vi "Reshaper1.vi"(3 "error IN":errorcluster, 5 "[IN] (X,Y,dX,dY)":dbl[][](array[numeric])) -> (0 "error OUT":errorcluster, 2 "[OUT] Reshaped (X,Y,dX,dY)":dbl[][](array[numeric]))   [LabVIEW 2017]
doc: "Deleting zero points in tracks (zero displacements)"
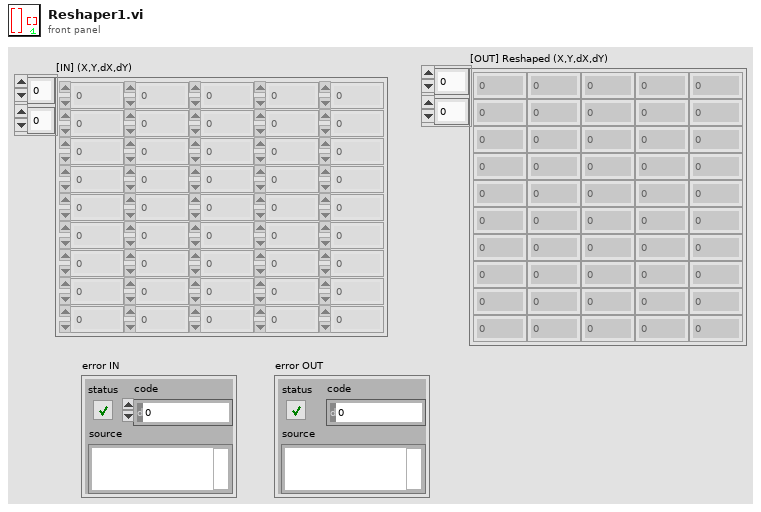
[diagram p1: front panel]
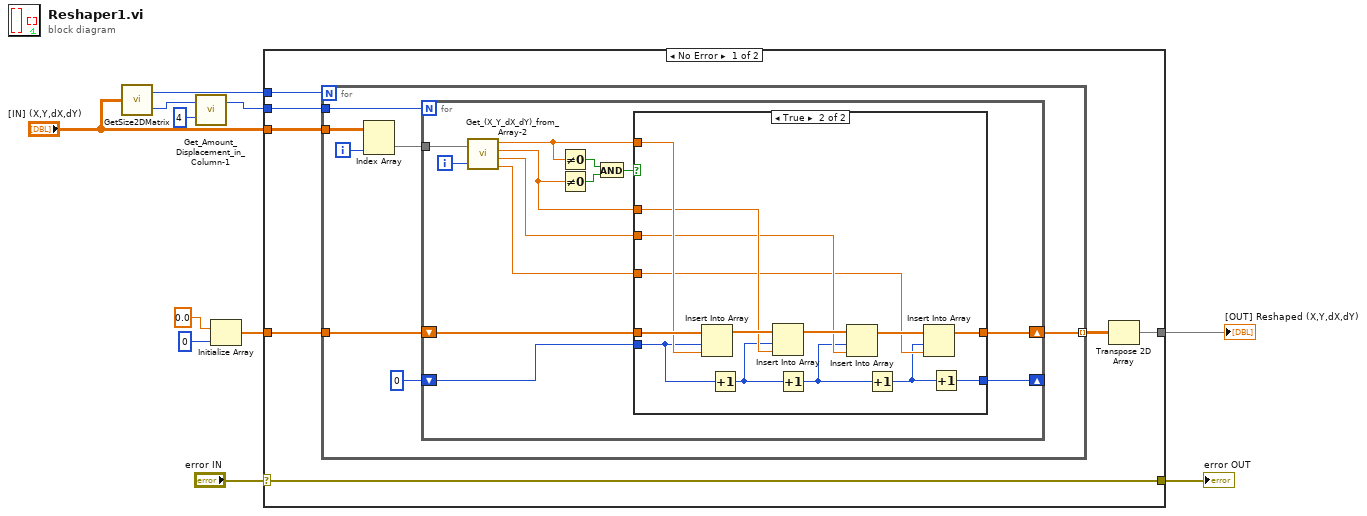
[diagram p0: block diagram]
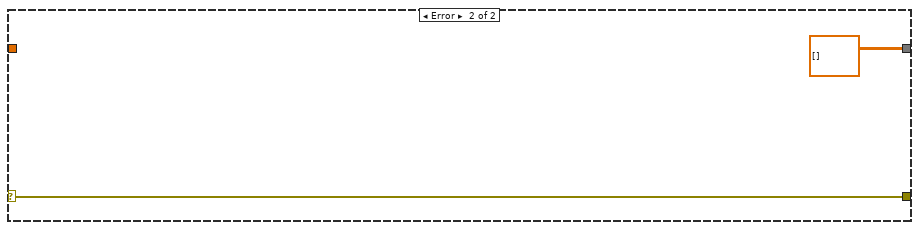
[diagram p3: hidden frame]
diagram:
  n1 = call "GetSize2DMatrix.vi"("Array IN (2D)"="[IN] (X,Y,dX,dY)") -> ("# Cols"=w6:i32, "# Rows"=w5:i32)
  n2 = call "Get_Amount_Displacement_in_Column-1.vi"("multiplier"=4, "# Rows"=w5) -> ("Displ amount"=w3:i32)  [unwired: 1 out]
  n3 = Initialize Array(0.0 ("element"), 0 ("dimension size")) -> (w9:dbl[])
  n4 = case shown="No Error" "error IN" {
    selector: "error IN" -> [w12 w55]
    tunnel: w9 -> [w18 _]
    tunnel: [w16 dbl[][] []] -> w8
    tunnel: "[IN] (X,Y,dX,dY)" -> [w15 _]
    tunnel: w6 -> [w14 _]
    tunnel: w3 -> [w13 _]
    tunnel: [w12 w55] -> w1
    frame No Error {
      n5 = for {
        N: w14 -> [_]
        tunnel: w15 -> [w25]
        tunnel: w18 -> [w22]
        tunnel: [w21] -> w17 mode=indexing
        tunnel: w13 -> [w19]
        i -> [w24]
        n6 = Index Array(array=w25, index (col)=w24) -> (element=w23:dbl[])  [unwired: 1 in]
        n7 = for {
          N: w19 -> [_]
          tunnel: w23 -> [w30]
          shift-right: [w34] -> w21
          shift-left: w22 -> [w35]
          shift-right: [w32] -> _
          shift-left: 0 -> [w33]
          i -> [w31]
          n8 = call "Get_(X_Y_dX_dY)_from_Array-2.vi"("(X,Y,dX,dY)"=w30, "Index of Displacement"=w31) -> ("X"=w29:dbl, "Y"=w28:dbl, "dX"=w27:dbl, "dY"=w26:dbl)
          n9 = Not Equal To 0?(x=w29) -> (x != 0?=w37:bool)
          n10 = Not Equal To 0?(x=w28) -> (x != 0?=w38:bool)
          n11 = And(x=w37, y=w38) -> (x .and. y?=w36:bool)
          n12 = case shown="True" w36 {
            tunnel: w35 -> [w40 w54]
            tunnel: w33 -> [w39 w52]
            tunnel: w29 -> [_ w53]
            tunnel: w28 -> [_ w50]
            tunnel: w27 -> [_ w48]
            tunnel: w26 -> [_ w45]
            tunnel: [w40 w43] -> w34
            tunnel: [w39 w41] -> w32
            frame False {
            }
            frame True {
              n13 = Insert Into Array(array=w54, index=w52, new element=w53) -> (w51:dbl[])
              n14 = Increment(x=w52) -> (x+1=w47:i32)
              n15 = Insert Into Array(array=w51, index=w47, new element=w50) -> (w49:dbl[])
              n16 = Increment(x=w47) -> (x+1=w44:i32)
              n17 = Insert Into Array(array=w49, index=w44, new element=w48) -> (w46:dbl[])
              n18 = Increment(x=w44) -> (x+1=w42:i32)
              n19 = Insert Into Array(array=w46, index=w42, new element=w45) -> (w43:dbl[])
              n20 = Increment(x=w42) -> (x+1=w41:i32)
            }
          }
        }
      }
      n21 = Transpose 2D Array(2D array=w17) -> (transposed array=w16:dbl[][])
    }
    frame Error {
    }
  }
  "[OUT] Reshaped (X,Y,dX,dY)" <- w8
  "error OUT" <- w1
